vi "SR_M-Save_Mission.vi"(11 "Mission In in":T1[](array[typedef]) {"GPS Longitude" format="%.6g"; "GPS Latitude" format="%.6g"}) -> (3 "Mission In out":T1[](array[typedef]) {"GPS Longitude" format="%.6g"; "GPS Latitude" format="%.6g"})   [LabVIEW 2015, in "Shore Library.lvlib"]
uses:
  Shore Library.lvlib
  RDS Mission Controller Actor/MissionOp.ctl
  RDS Mission Controller Actor/RDS Mission Controller Actor.lvlib
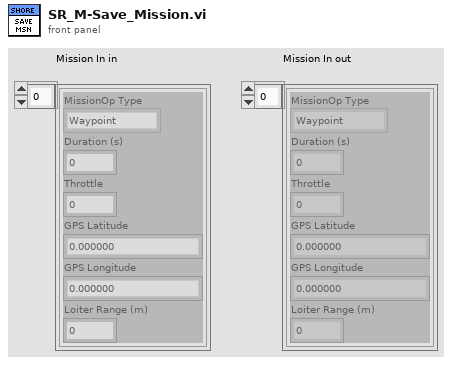
[diagram p1: front panel]
types:
  T1 = typedef "RDS Mission Controller Actor.lvlib/MissionOp.ctl" = cluster{"MissionOp Type":enum16{"Waypoint", "Loiter", "Wait", "Deploy AIP", "Stow AIP"}, "Duration (s)":u16, "Throttle":i16, "GPS Latitude":dbl, "GPS Longitude":dbl, "Loiter Range (m)":u16}
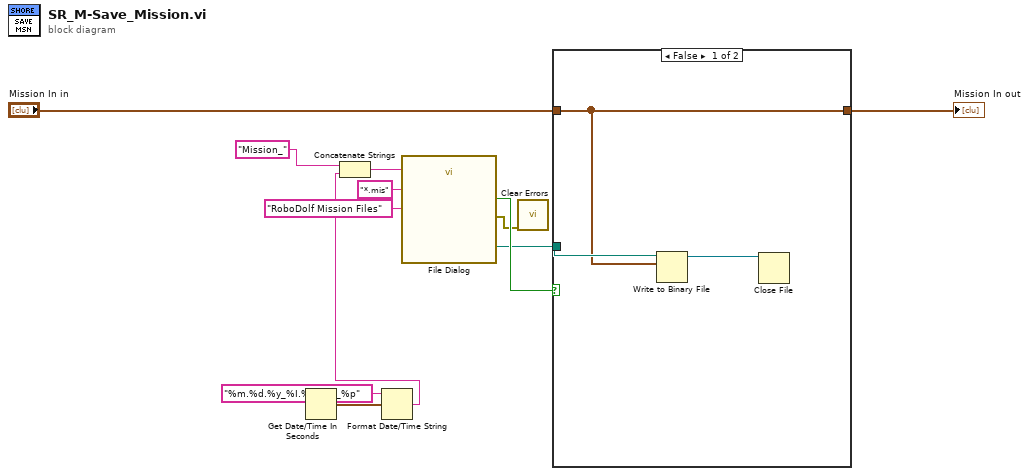
[diagram p0: block diagram]
diagram:
  n1 = Get Date/Time In Seconds() -> (seconds since 1Jan1904=w2:timestamp)
  n2 = Format Date/Time String(time format string (%c)="%m.%d.%y_%I.%M.%S_%p", seconds (now)=w2) -> (date/time string=w5:string)  [unwired: 1 in]
  n3 = Concatenate Strings("Mission_" ("default name"), w5) -> (w6:string)
  n4 = call "File Dialog"("default name"=w6, "pattern (all files)"="*.mis", "pattern label"="RoboDolf Mission Files") -> ("selected path"=w7:path, "cancelled"=w9:bool, "error out"=w8:errorcluster)  [unwired: 9 in, 1 out]
  n5 = call <vilib>:"Clear Errors.vi"("error in (no error)"=w8) -> ()  [unwired: 5 in, 2 out]
  n6 = case shown="False" w9 {
    tunnel: w7 -> [w15 _]
    tunnel: "Mission In in" -> [w13 w16]
    tunnel: [w13 w16] -> w11
    frame False {
      n7 = Write to Binary File(file (use dialog)=w15, data=w13) -> (refnum out=w14:refnum<file>)  [unwired: 4 in, 2 out]
      n8 = Close File(refnum=w14) -> ()  [unwired: 1 in, 2 out]
    }
    frame True {
    }
  }
  "Mission In out" <- w11
